vi "Actor Core.vi"(8 "error in":errorcluster, 11 "Nested in":refnum<class "[V] Sys Cfg Main.lvclass">) -> (0 "error out":errorcluster, 3 "Actor out":refnum<class "Actor.lvclass">)   [LabVIEW 2020, in "[V] Sys Cfg Main.lvlib" / "[V] Sys Cfg Main.lvclass"]
doc: "(<B>Filename</B>: Actor Framework.lvlib:Actor.lvclass:Actor Core.vi)\n\nReceives messages to the actor, reacts to them, and initiates any error handling that may shut the actor down.\n\nDescendant classes may override this VI to append parallel tasks for the actor to complete while it handles messages. Overrides use the Call Parent Method node."
uses:
  [V] Sys Cfg Main.lvclass
  C:/Program Files (x86)/National Instruments/LabVIEW 2020/vi.lib/ActorFramework/Actor/Actor.lvclass
  <vilib>/ActorFramework/Actor/Actor.lvclass
  <vilib>/ActorFramework/Actor/Actor.lvclass/Actor.ctl
  <vilib>/ActorFramework/Message Enqueuer/Message Enqueuer.lvclass/Message Enqueuer.ctl
  [V] Sys Cfg Main.lvclass/[V] Sys Cfg Main.ctl
  [V] Sys Cfg Main Messages/Event Tree Msg/Event Tree Msg.lvclass/Event Tree Msg.ctl
  <vilib>/ActorFramework/Message Enqueuer/Init from Existing Queue.vi
  <vilib>/ActorFramework/Message Enqueuer/Enqueue.vi
  [V] Sys Cfg Main Messages/Event Tree Msg/Event Tree Msg.lvclass
  C:/Program Files (x86)/National Instruments/LabVIEW 2020/vi.lib/ActorFramework/Message/Message.lvclass
  [V] Sys Cfg Main Messages/Event Comfirm Msg/Event Comfirm Msg.lvclass
  [V] Sys Cfg Main Messages/Event Apply Msg/Event Apply Msg.lvclass
  <vilib>/ActorFramework/Stop Msg/Stop Msg.lvclass
  <vilib>/ActorFramework/Message Priority Queue/Priority Enqueue.vi
  <vilib>/ActorFramework/Message Enqueuer/Message Enqueuer.lvclass
panel:
  in  "tree":string(tree)
  in  "cancel":bool
  in  "apply":bool
  in  "confirm":bool
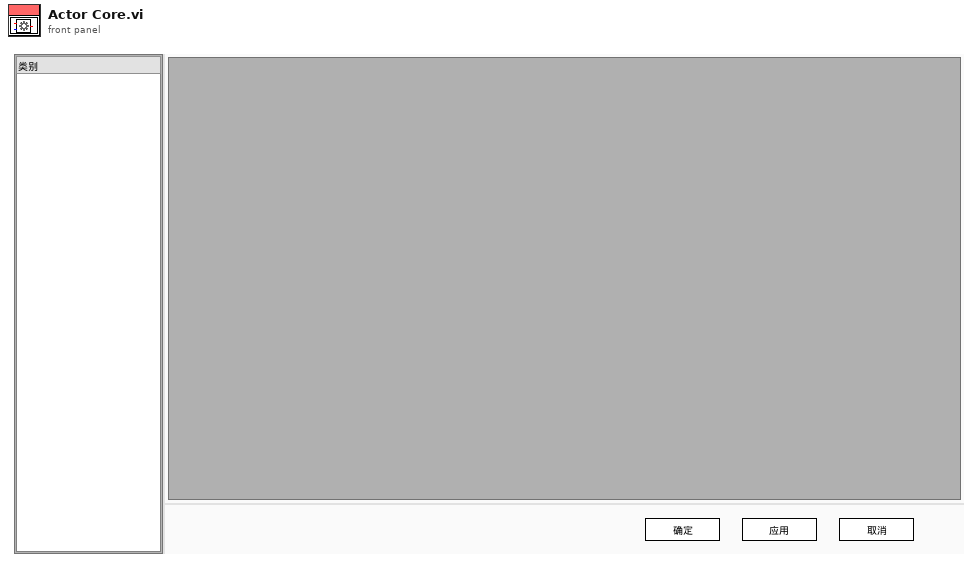
[diagram p1: front panel]
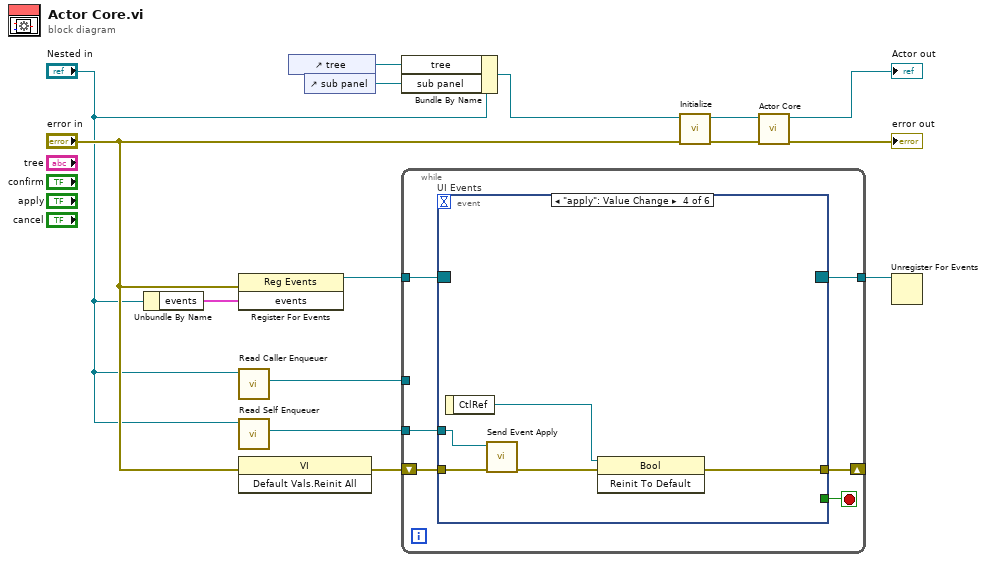
[diagram p0: block diagram]
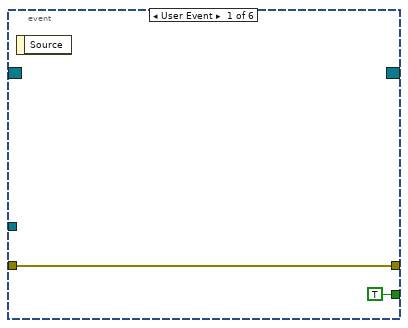
[diagram p2: hidden frame]
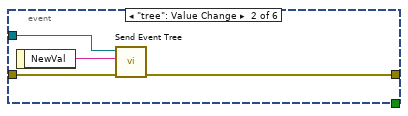
[diagram p3: hidden frame]
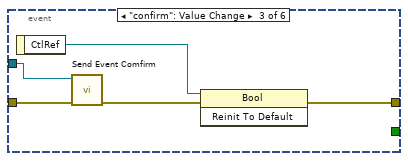
[diagram p4: hidden frame]
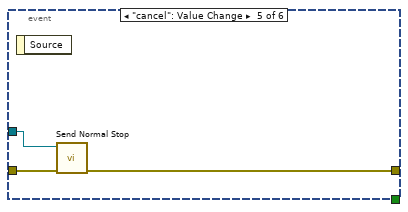
[diagram p5: hidden frame]
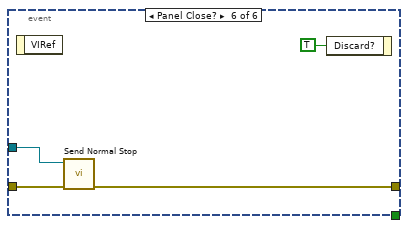
[diagram p6: hidden frame]
diagram:
  n1 = Unbundle By Name("Nested in") -> ("events"=w12:cluster{"stop":refnum<user-event>})
  n2 = register-events ("Main Register for Events")(error in="error in", w12) -> (reference out=w13:refnum<event-registration>)  [unwired: 1 in, 1 out]
  n3 = call <vilib>:"Read Caller Enqueuer.vi"("Actor"="Nested in") -> ("Caller Enqueuer"=w9:refnum<class "Message Enqueuer.lvclass">)  [unwired: 10 in]
  n4 = call <vilib>:"Read Self Enqueuer.vi"("Actor"="Nested in") -> ("Self Enqueuer"=w10:refnum<class "Message Enqueuer.lvclass">)  [unwired: 10 in]
  n5 = invoke class="VI" method="Default Vals.Reinit All"(error in="error in") -> (error out=w8:errorcluster)  [unwired: 2 in, 2 out]
  n6 = control-ref of="tree"() -> (w1:refnum<vi>)
  n7 = control-ref of="sub panel"() -> (w2:refnum<vi>)
  n8 = Bundle By Name(cluster="Nested in", "tree"=w1, "sub panel"=w2) -> (w3:refnum<class "[V] Sys Cfg Main.lvclass">)
  n9 = while {
    tunnel: w13 -> [w21]
    tunnel: [w19] -> w11
    tunnel: w10 -> [w18]
    tunnel: w9 -> [_]
    shift-right: [w16] -> _
    shift-left: w8 -> [w17]
    stop <- w20 stop-if-true
    n10 = event "UI Events" shown="[3] \"apply\": Value Change" {
      selector: w21 -> [_ _ _ _ _ _]
      dyn-events: [_ _ _ _ _ _] -> w19
      timeout: _ -> [_ _ _ _ _ _]
      tunnel: [TRUE _ _ _ _ _] -> w20
      tunnel: w18 -> [_ w26 w31 w36 w38 w43]
      tunnel: w17 -> [w23 w27 w32 w37 w40 w42]
      tunnel: [w23 w25 w29 w33 w39 w41] -> w16
      event User Event {
        n11 = event-data() -> ()  [unwired: 1 in, 1 out]
      }
      event "tree": Value Change {
        n12 = event-data() -> ("NewVal"=w24:string)  [unwired: 1 in]
        n13 = call "Send Event Tree.vi"("error in (no error)"=w27, "item"=w24, "Message Enqueuer"=w26) -> ("error out"=w25:errorcluster)  [unwired: 7 in, 1 out]
      }
      event "confirm": Value Change {
        n14 = event-data() -> ("CtlRef"=w28:refnum<vi>)  [unwired: 1 in]
        n15 = call "Send Event Comfirm.vi"("error in (no error)"=w32, "Message Enqueuer"=w31) -> ("error out"=w30:errorcluster)  [unwired: 8 in, 1 out]
        n16 = invoke class="Bool" method="Reinit To Default"(reference=w28, error in=w30) -> (error out=w29:errorcluster)  [unwired: 1 in, 2 out]
      }
      event "apply": Value Change {
        n17 = event-data() -> ("CtlRef"=w35:refnum<vi>)  [unwired: 1 in]
        n18 = call "Send Event Apply.vi"("error in (no error)"=w37, "Message Enqueuer"=w36) -> ("error out"=w34:errorcluster)  [unwired: 8 in, 1 out]
        n19 = invoke class="Bool" method="Reinit To Default"(reference=w35, error in=w34) -> (error out=w33:errorcluster)  [unwired: 1 in, 2 out]
      }
      event "cancel": Value Change {
        n20 = event-data() -> ()  [unwired: 1 in, 1 out]
        n21 = call <vilib>:"Send Normal Stop.vi"("error in (no error)"=w40, "Message Enqueuer"=w38) -> ("error out"=w39:errorcluster)  [unwired: 9 in]
      }
      event Panel Close? {
        n22 = event-data() -> ()  [unwired: 1 in, 1 out]
        n23 = call <vilib>:"Send Normal Stop.vi"("error in (no error)"=w42, "Message Enqueuer"=w43) -> ("error out"=w41:errorcluster)  [unwired: 9 in]
        n24 = event-data("Discard?"=TRUE) -> ()  [unwired: 1 in, 1 out]
      }
    }
  }
  n25 = call "Initialize.vi"("error in (no error)"="error in", "View Template in"=w3) -> ("error out"=w7:errorcluster, "View Template out"=w6:refnum<class "[V] Sys Cfg Main.lvclass">)  [unwired: 8 in]
  n26 = call-parent "Actor Core.vi"("error in"=w7, "Actor in"=w6) -> ("error out"=→"error out":errorcluster, "Actor out"=→"Actor out":refnum<class "Actor.lvclass">)  [unwired: 8 in]
  n27 = Unregister For Events(event registration refnum=w11) -> ()  [unwired: 1 in, 1 out]
